vi "task2.2_better.vi"() -> ()   [LabVIEW 2021]
doc: "This example demonstrates how to continuously re-generate analog output data from a buffer in your computer's memory.\n\nRefer to your device documentation for pinouts and hardware capabilities."
uses:
  <vilib>/DAQmx/write.llb/DAQmx Write (Analog Wfm 1Chan NSamp).vi
  <vilib>/DAQmx/write.llb/DAQmx Write (Digital Bool 1Line 1Point).vi
  <vilib>/DAQmx/read.llb/DAQmx Read (Analog 1D Wfm NChan NSamp).vi
  <vilib>/DAQmx/create/channels.llb/DAQmx Create Channel (AO-Voltage-Basic).vi
  <vilib>/DAQmx/configure/timing.llb/DAQmx Timing (Sample Clock).vi
  <vilib>/DAQmx/create/channels.llb/DAQmx Create Channel (AI-Voltage-Basic).vi
  <vilib>/DAQmx/configure/trigger.llb/DAQmx Start Trigger (Digital Edge).vi
  <vilib>/DAQmx/miscellaneous.llb/DAQmx Fill In Error Info.vi
  <vilib>/DAQmx/create/channels.llb/DAQmx Create Channel (DO-Digital Output).vi
  <vilib>/Waveform/WDTFileIO.llb/ Write Waveform to File.vi
  <vilib>/Waveform/WDTFileIO.llb/ Write Waveforms to File (1D).vi
  <vilib>/express/express analysis/Spectral/Block/exnSpectralBlock spectral measurements peak poly.vi
  <vilib>/express/express analysis/Spectral/Block/exnSpectralBlock spectral measurements peak array WFM.vi
  <vilib>/express/express analysis/Spectral/Block/exnSpectralBlock spectral measurements peak WFM.vi
  <vilib>/express/express analysis/Spectral/XNode/ExpressSpectralMeasurementsBlockNode.xnode
  <vilib>/measure/NI_MABase.lvlib
panel:
  out "Output Freq":cluster{"f0":dbl, "df":dbl, "magnitude":dbl[]}(graph)
  out "Input Freq":cluster{"f0":dbl, "df":dbl, "magnitude":dbl[]}[](graph)
  in  "Amplitude":dbl=1.0 format="%0.2p"
  in  "Frequency":dbl=10.0 format="%0.2p"
  in  "Waveform Type":u16(ring) items=["Sine Wave", "Triangle Wave", "Square Wave", "Sawtooth Wave"]
  in  "Input Channel 2":tag="Dev3/ai1"
  in  "Number of samples":i32=1000
  out "Input Voltage":waveform(dbl)[](graph)=[{"t0"=timestamp(3702416907.610318 s since 1904-01-01), "dt"=9.999999999999999e-05, "Y"=array[1000 elements], "attributes"=variant("NI_ChannelName"=variant(string "Dev6/ai0"), "NI_UnitDescription"=variant(string "Volts"))}, {"t0"=timestamp(3702416907.610332 s since 1904-01-01), "dt"=9.999999999999999e-05, "Y"=array[1000 elements], "attributes"=variant("NI_ChannelName"=variant(string "Dev6/ai1"), "NI_UnitDescription"=variant(string "Volts"))}]
  in  "Input Channel 1":tag="Dev3/ai0"
  in  "Min Input Voltage":dbl=-10.0
  in  "Max Input Voltage":dbl=10.0
  in  "Output sample rate":dbl=10000.0 format="%0.2f"
  out "Output Voltage":waveform(dbl)(graph)={"t0"=timestamp(0 s since 1904-01-01), "dt"=0.0001, "Y"=array[1000 elements]}
  in  "Max Voltage":dbl=10.0
  in  "Min Voltage":dbl=-10.0
  in  "Output Channel":tag="Dev3/ao0"
  # "Output Channel Settings"
  # "Output voltage"
  # "Input voltage"
  # "Input Channel Settings"
  # "Waveform Settings"
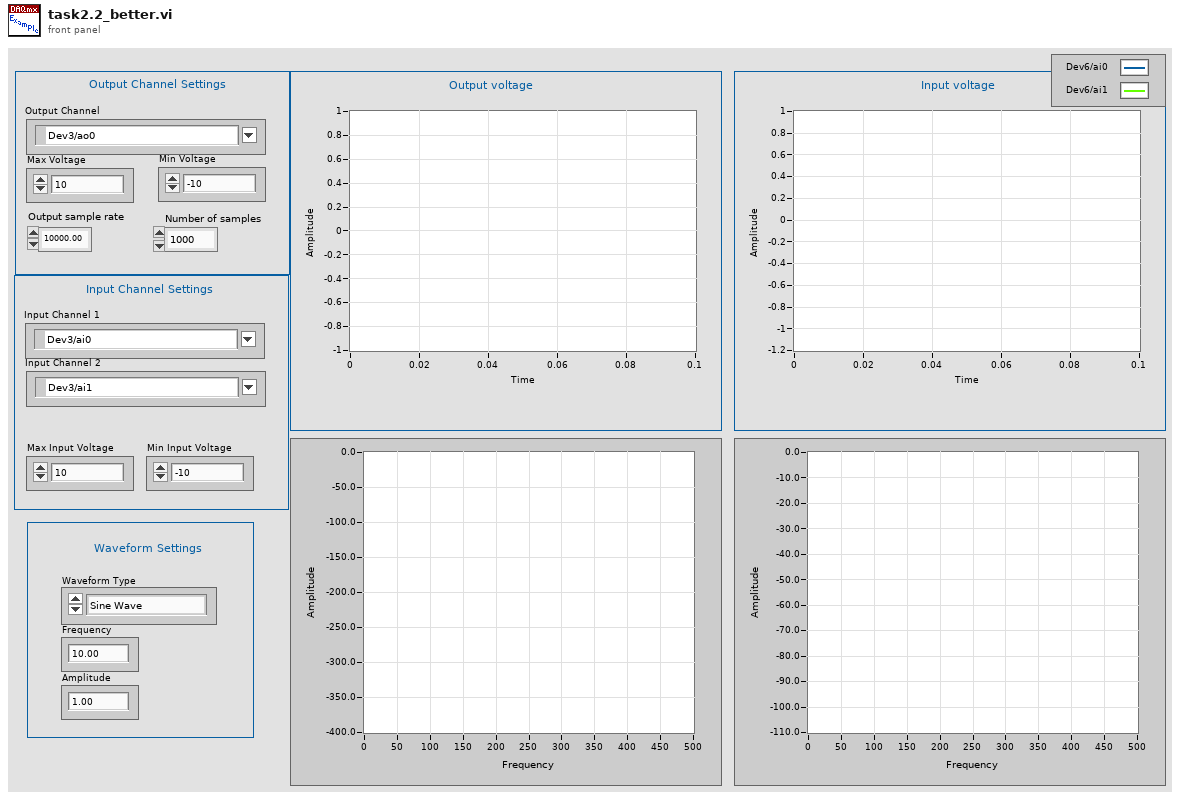
[diagram p1: front panel]
types:
  T1 = cluster{"Output sample rate":dbl, "Number of samples":i32}
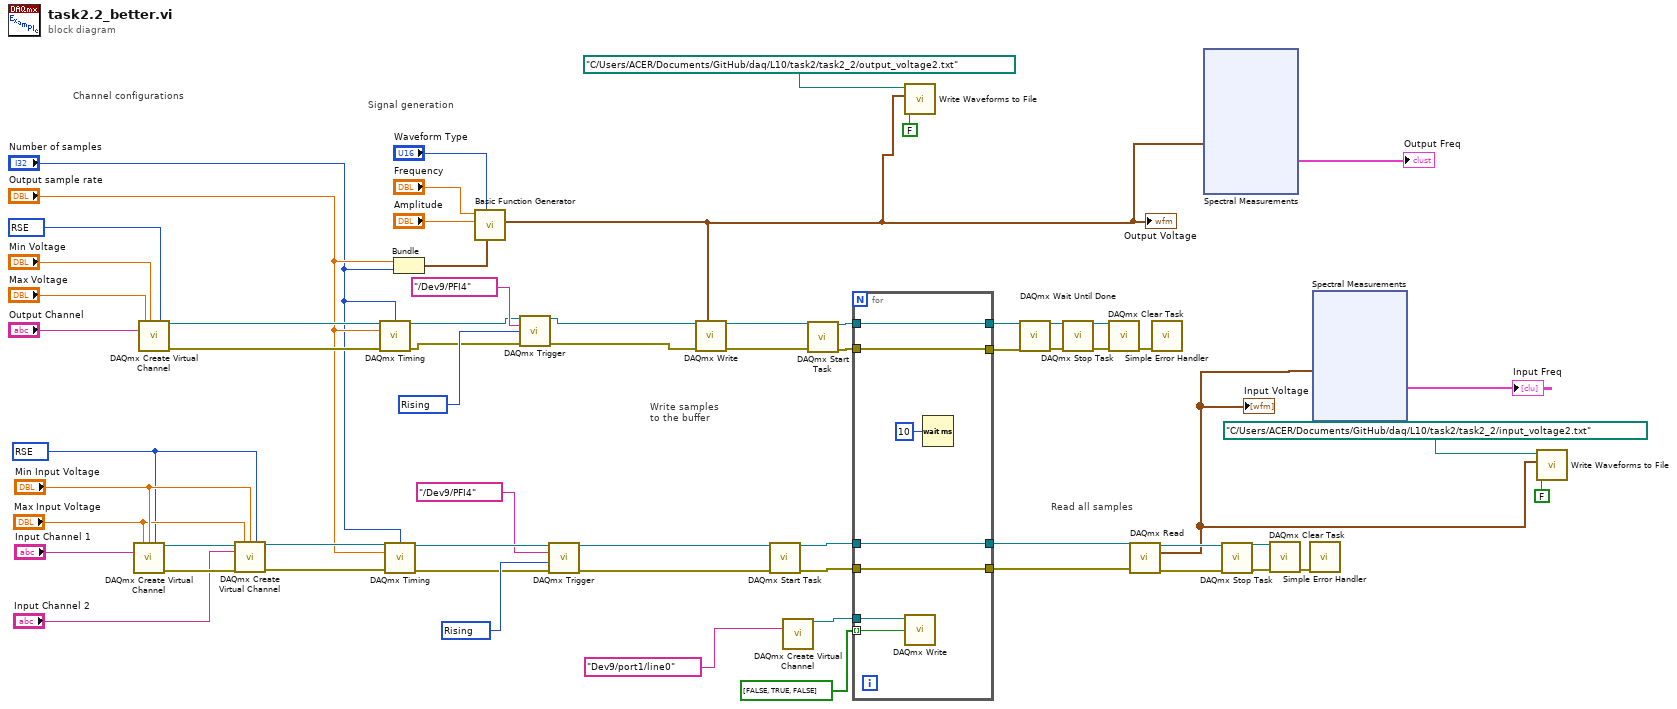
[diagram p0: block diagram]
diagram:
  w11 = 10280 items=["Rising"=10280, "Falling"=10171] ("edge")
  w15 = 10280 items=["Rising"=10280, "Falling"=10171] ("edge")
  w39 = 10083 items=["Default"=-1, "RSE"=10083, "NRSE"=10078, "Differential"=10106, "Pseudodifferential"=12529] ("input terminal configuration")
  w53 = 10083 items=["Default"=-1, "RSE"=10083, "NRSE"=10078, "Differential"=10106, "Pseudodifferential"=12529] ("input terminal configuration")
  # "Read all samples"
  # "Write samples\nto the buffer"
  # "Signal generation"
  # "Channel configurations"
  n1 = call-poly <vilib>:"DAQmx Create Virtual Channel.vi"("maximum value"="Max Input Voltage", "minimum value"="Min Input Voltage", "input terminal configuration"=w39, "physical channels"="Input Channel 1") -> ("task out"=w49:refnum<k21>, "error out"=w50:errorcluster)  [unwired: 10 in]
  n2 = call-poly <vilib>:"DAQmx Create Virtual Channel.vi"("maximum value"="Max Voltage", "minimum value"="Min Voltage", "output terminal configuration"=w53, "physical channels"="Output Channel") -> ("task out"=w57:refnum<k21>, "error out"=w58:errorcluster)  [unwired: 10 in]
  n3 = call-poly <vilib>:"DAQmx Create Virtual Channel.vi"("task in"=w49, "maximum value"="Max Input Voltage", "minimum value"="Min Input Voltage", "input terminal configuration"=w39, "physical channels"="Input Channel 2", "error in"=w50) -> ("task out"=w48:refnum<k21>, "error out"=w47:errorcluster)  [unwired: 8 in]
  n4 = call-poly <vilib>:"DAQmx Timing.vi"("task/channels in"=w57, "samples per channel"="Number of samples", "rate"="Output sample rate", "error in"=w58) -> ("task out"=w16:refnum<k21>, "error out"=w14:errorcluster)  [unwired: 10 in]
  n5 = call-poly <vilib>:"DAQmx Timing.vi"("task/channels in"=w48, "samples per channel"="Number of samples", "rate"="Output sample rate", "error in"=w47) -> ("task out"=w8:refnum<k21>, "error out"=w10:errorcluster)  [unwired: 10 in]
  n6 = Bundle "Bundle"("Output sample rate"="Output sample rate", "Number of samples"="Number of samples") -> (w38:T1)  [unwired: 1 in]
  n7 = call <vilib>:"Basic Function Generator.vi"("sampling info"=w38, "signal type"="Waveform Type", "amplitude"="Amplitude", "frequency"="Frequency") -> ("signal out"=w1:waveform(dbl))  [unwired: 5 in, 2 out]
  "Output Voltage" <- w1
  n8 = call-poly <vilib>:"DAQmx Trigger.vi"("task/channels in"=w16, "source"=tag "/Dev9/PFI4", "edge"=w15, "error in"=w14) -> ("task out"=w19:refnum<k21>, "error out"=w18:errorcluster)  [unwired: 10 in]
  n9 = call-poly <vilib>:"DAQmx Trigger.vi"("task/channels in"=w8, "source"=tag "/Dev9/PFI4", "edge"=w11, "error in"=w10) -> ("task out"=w13:refnum<k21>, "error out"=w12:errorcluster)  [unwired: 10 in]
  n10 = call-poly <vilib>:"DAQmx Write.vi"("task/channels in"=w19, "data"=w1, "error in"=w18) -> ("task out"=w21:refnum<k21>, "error out"=w20:errorcluster)  [unwired: 10 in, 1 out]
  n11 = call <vilib>:"DAQmx Start Task.vi"("task/channels in"=w13, "error in"=w12) -> ("task out"=w28:refnum<k21>, "error out"=w29:errorcluster)  [unwired: 12 in]
  n12 = call-poly <vilib>:"DAQmx Create Virtual Channel.vi"("lines"=tag "Dev9/port1/line0") -> ("task out"=w26:refnum<k21>)  [unwired: 13 in, 1 out]
  n13 = call <vilib>:"DAQmx Start Task.vi"("task/channels in"=w21, "error in"=w20) -> ("task out"=w30:refnum<k21>, "error out"=w31:errorcluster)  [unwired: 12 in]
  n14 = for {
    tunnel: bool[] [FALSE, TRUE, FALSE] -> [w70] mode=indexing
    tunnel: w29 -> [w66]
    tunnel: w28 -> [w67]
    tunnel: w31 -> [w68]
    tunnel: w30 -> [w69]
    tunnel: [w69] -> w25
    tunnel: [w68] -> w24
    tunnel: [w67] -> w23
    tunnel: [w66] -> w22
    tunnel: w26 -> [w65]
    n15 = call-poly <vilib>:"DAQmx Write.vi"("task/channels in"=w65, "data"=w70) -> ()  [unwired: 11 in, 3 out]
    n16 = Wait (ms)(milliseconds to wait=u32 10) -> ()  [unwired: 1 out]
  }
  n17 = call-poly <vilib>:"Write Waveforms to File.vi"("append to file? (new file:F)"=FALSE, "waveform"=w1, "file path (dialog if empty)"=path "C:/Users/ACER/Documents/GitHub/daq/L10/task2/task2_2/output_voltage2.txt") -> ()  [unwired: 7 in, 2 out]
  n18 = call <vilib>:"DAQmx Wait Until Done.vi"("task/channels in"=w25, "error in"=w24) -> ("task out"=w35:refnum<k21>, "error out"=w34:errorcluster)  [unwired: 12 in]
  n19 = call <vilib>:"DAQmx Stop Task.vi"("task/channels in"=w35, "error in"=w34) -> ("task out"=w60:refnum<k21>, "error out"=w59:errorcluster)  [unwired: 12 in]
  n20 = call <vilib>:"DAQmx Clear Task.vi"("task in"=w60, "error in"=w59) -> ("error out"=w64:errorcluster)  [unwired: 13 in]
  n21 = call-poly <vilib>:"DAQmx Read.vi"("task/channels in"=w23, "error in"=w22) -> ("task out"=w51:refnum<k21>, "data"=w2:waveform(dbl)[], "error out"=w52:errorcluster)  [unwired: 11 in]
  "Input Voltage" <- w2
  n22 = call <vilib>:"Simple Error Handler.vi"("error in (no error)"=w64) -> ()  [unwired: 4 in, 5 out]
  n23 = xnode "Spectral Measurements"("Signals"=w1) -> ("FFT - (Peak)"=→"Output Freq":cluster{"f0":dbl, "df":dbl, "magnitude":dbl[]})  [unwired: 1 in, 2 out]
  n24 = call <vilib>:"DAQmx Stop Task.vi"("task/channels in"=w51, "error in"=w52) -> ("task out"=w55:refnum<k21>, "error out"=w56:errorcluster)  [unwired: 12 in]
  n25 = call <vilib>:"DAQmx Clear Task.vi"("task in"=w55, "error in"=w56) -> ("error out"=w54:errorcluster)  [unwired: 13 in]
  n26 = call <vilib>:"Simple Error Handler.vi"("error in (no error)"=w54) -> ()  [unwired: 4 in, 5 out]
  n27 = xnode "Spectral Measurements"("Signals"=w2) -> ("FFT - (Peak)"=→"Input Freq":cluster{"f0":dbl, "df":dbl, "magnitude":dbl[]}[])  [unwired: 1 in, 2 out]
  n28 = call-poly <vilib>:"Write Waveforms to File.vi"("append to file? (new file:F)"=FALSE, "waveform array"=w2, "file path (dialog if empty)"=path "C:/Users/ACER/Documents/GitHub/daq/L10/task2/task2_2/input_voltage2.txt") -> ()  [unwired: 7 in, 2 out]
